vi "校准设置页.vi"() -> ()   [LabVIEW 2016, in "斯坦道总磷.lvlib"]
uses:
  <vilib>/ptbypt/NI_PtbyPt.lvlib
panel:
  in  "校准任务":bool
  in  "历史数据导入":T1(radio)
  out "刷新时间":string
  out "模型刷新":bool
  in  "校准按钮":T1(radio)
  in  "仪器写入":bool
  in  "辅助计算":bool
  in  "曲线模型":T2={"标液浓度1"=0.0, "测量吸光度1"=0.0, "样品1启用"=FALSE, "标液浓度2"=0.0, "测量吸光度2"=0.0, "样品2启用"=FALSE, "标液浓度3"=0.0, "测量吸光度3"=0.0, "样品3启用"=FALSE, "标液浓度4"=0.0, "测量吸光度4"=0.0, "样品4启用"=FALSE, "标液浓度5"=0.0, "测量吸光度5"=0.0, "样品5启用"=FALSE, "模型"=enum."线性", "精度"=4.0, "XY图"=[], "拟合公式"="", "r^2"=0.0, "标样一校准时间"=timestamp(0 s since 1904-01-01), "标样二校准时间"=timestamp(0 s since 1904-01-01), "标样三校准时间"=timestamp(0 s since 1904-01-01), "标样四校准时间"=timestamp(0 s since 1904-01-01), "标样五校准时间"=timestamp(0 s since 1904-01-01), "二次方程"={"c"=0.0, "x"=0.0, "x^2"=0.0}, "标定时间"=timestamp(0 s since 1904-01-01)} {"标定时间" format="%<%y/%m/%d %H:%M:%S>T"; "标样五校准时间" format="%<%y/%m/%d %H:%M:%S>T"; "标样四校准时间" format="%<%y/%m/%d %H:%M:%S>T"; "标样三校准时间" format="%<%y/%m/%d %H:%M:%S>T"; "标样二校准时间" format="%<%y/%m/%d %H:%M:%S>T"; "标样一校准时间" format="%<%y/%m/%d %H:%M:%S>T"; "r^2" format="%.7f"; "测量吸光度5" format="%#.6f"; "测量吸光度4" format="%#.6f"; "测量吸光度3" format="%#.6f"; "测量吸光度2" format="%#.6f"; "测量吸光度1" format="%#.6f"}
  in  "测量模式":T3(ring)
  in  "参数下拉列表":u16(ring)
  in  "量程下拉列表":enum16{"低量程", "高量程"}(ring)
  # "校准时间"
  # "标液浓度"
  # "吸光值"
  # "标样一"
  # "标样二"
  # "标样三"
  # "零点"
  # "跨度"
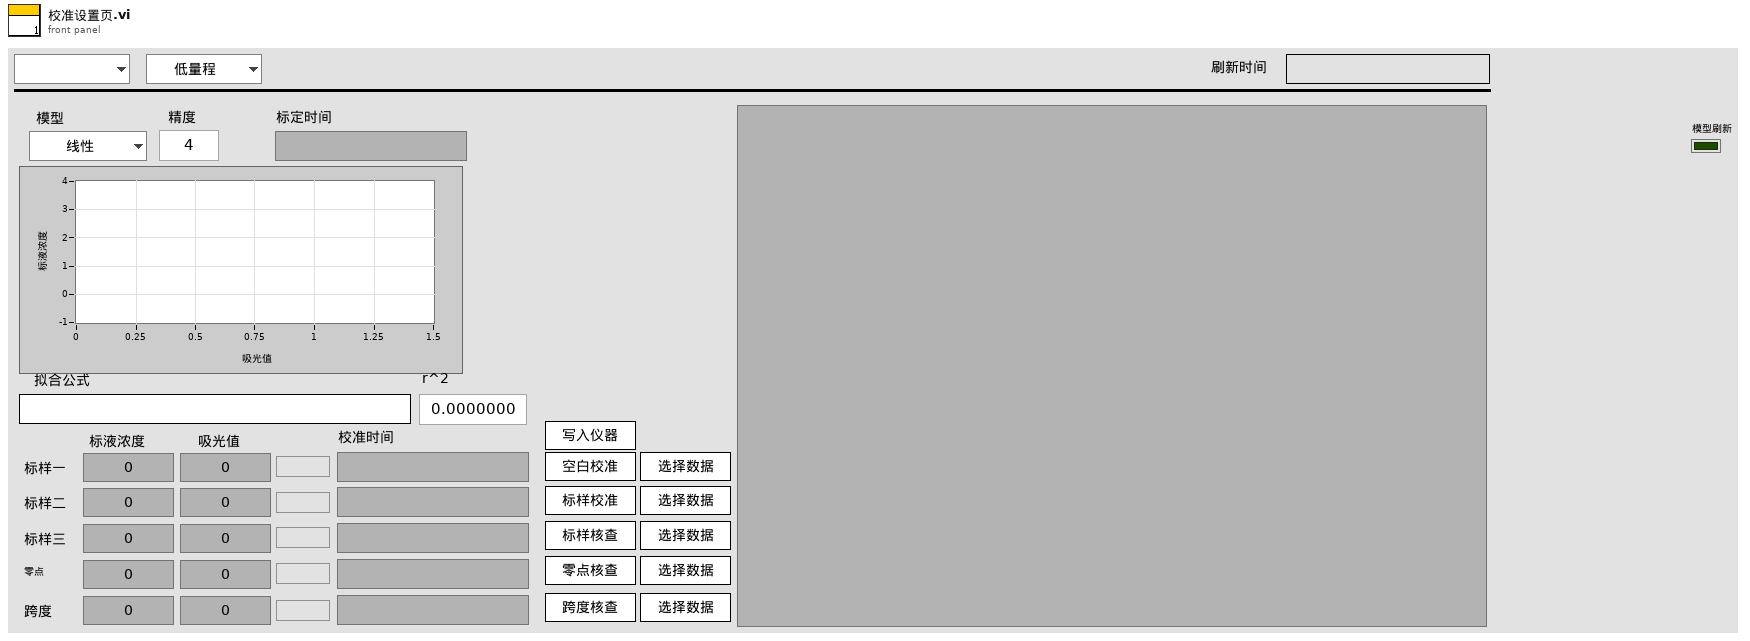
[diagram p1: front panel]
types:
  T1 = enum32{"未选择", "空白校准", "标样校准", "标样核查", "零点核查", "跨度核查"}
  T2 = cluster{"标液浓度1":dbl, "测量吸光度1":dbl, "样品1启用":bool, "标液浓度2":dbl, "测量吸光度2":dbl, "样品2启用":bool, "标液浓度3":dbl, "测量吸光度3":dbl, "样品3启用":bool, "标液浓度4":dbl, "测量吸光度4":dbl, "样品4启用":bool, "标液浓度5":dbl, "测量吸光度5":dbl, "样品5启用":bool, "模型":enum32{"线性", "多项式"}, "精度":dbl, "XY图":cluster{"X Values":dbl[], "Y Values":dbl[]}[], "拟合公式":string, "r^2":dbl, "标样一校准时间":timestamp, "标样二校准时间":timestamp, "标样三校准时间":timestamp, "标样四校准时间":timestamp, "标样五校准时间":timestamp, "二次方程":cluster{"c":dbl, "x":dbl, "x^2":dbl}, "标定时间":timestamp}
  T3 = enum16{"跨度核查", "水样测量", "零点核查", "标样核查", "加标回收", "快捷测试", "空白校准", "标样校准"}
  T4 = typedef "斯坦道总磷.lvlib/校准任务.ctl" = cluster{"id":u16, "任务类型":enum16{"未选择", "空白校准", "标样校准", "标样核查", "零点核查", "跨度核查"}, "量程下拉列表":enum16{"低量程", "高量程"}, "状态":enum16{"已执行", "待执行", "执行中", "停止"}, "标液浓度":dbl, "吸光值":dbl, "校准时间":timestamp}
  T5 = enum8{"Enabled", "Disabled", "Disabled and Grayed Out"}
  T6 = cluster{"低标液1浓度":dbl, "低标液1信号值":dbl, "低标液1启用":u16, "低标液2浓度":dbl, "低标液2信号值":dbl, "低标液2启用":u16, "低标液3浓度":dbl, "低标液3信号值":dbl, "低标液3启用":u16, "低标液4浓度":dbl, "低标液4信号值":dbl, "低标液4启用":u16, "低标液5浓度":dbl, "低标液5信号值":dbl, "低标液5启用":u16, "高标液1浓度":dbl, "高标液1信号值":dbl, "高标液1启用":u16, "高标液2浓度":dbl, "高标液2信号值":dbl, "高标液2启用":u16, "高标液3浓度":dbl, "高标液3信号值":dbl, "高标液3启用":u16, "高标液4浓度":dbl, "高标液4信号值":dbl, "高标液4启用":u16, "高标液5浓度":dbl, "高标液5信号值":dbl, "高标液5启用":u16}
  T7 = cluster{"标液浓度1":dbl, "测量吸光度1":dbl, "样品1启用":bool, "标液浓度2":dbl, "测量吸光度2":dbl, "样品2启用":bool, "标液浓度3":dbl, "测量吸光度3":dbl, "样品3启用":bool, "标液浓度4":dbl, "测量吸光度4":dbl, "样品4启用":bool, "标液浓度5":dbl, "测量吸光度5":dbl, "样品5启用":bool, "模型":enum32{"线性", "多项式"}, "精度":dbl, "XY图":cluster{"X Values":dbl[], "Y Values":dbl[]}[], "拟合公式":string, "r^2":dbl, "标样一校准时间":timestamp, "标样二校准时间":timestamp, "标样三校准时间":timestamp, "标样四校准时间":timestamp, "标样五校准时间":timestamp, "二次方程":cluster{"c":dbl, "x":dbl, "x^2":dbl}, "标定时间":timestamp}[]
  T8 = cluster{"标液浓度1":dbl, "测量吸光度1":dbl, "样品1启用":bool, "标液浓度2":dbl, "测量吸光度2":dbl, "样品2启用":bool, "标液浓度3":dbl, "测量吸光度3":dbl, "样品3启用":bool, "标液浓度4":dbl, "测量吸光度4":dbl, "样品4启用":bool, "标液浓度5":dbl, "测量吸光度5":dbl, "样品5启用":bool, "模型":enum32{"线性", "多项式"}, "精度":dbl, "XY图":cluster{"X Values":dbl[], "Y Values":dbl[]}[], "拟合公式":string, "r^2":dbl, "标样一校准时间":timestamp, "标样二校准时间":timestamp, "标样三校准时间":timestamp, "标样四校准时间":timestamp, "标样五校准时间":timestamp, "二次方程":cluster{"c":dbl, "x":dbl, "x^2":dbl}, "标定时间":timestamp}[][]
  T9 = typedef "LVStringsAndValuesArrayTypeDef_U16.ctl" = cluster{"String":string, "Value":u16}[]
  T10 = cluster{"系统时间":timestamp, "工作状态":u16, "测量模式":enum16{"待机", "连续模式", "周期模式", "定点模式", "受控模式", "手动模式"}, "告警代码":u16, "故障代码":u16, "日志代码":u16, "软件版本":u16, "F0":sgl, "F1":sgl, "F2":sgl, "F3":sgl, "T":sgl, "H":sgl, "id":u16, "flowid":u16, "量程":u16, "总磷控温温度1":sgl, "营养盐控温温度2":sgl, "ADC":sgl}
  T11 = cluster{"时间":timestamp, "标液值":dbl, "检测值":dbl, "吸光值":dbl}
  T12 = enum32{"Bad", "Idle", "Run top level", "Running"}
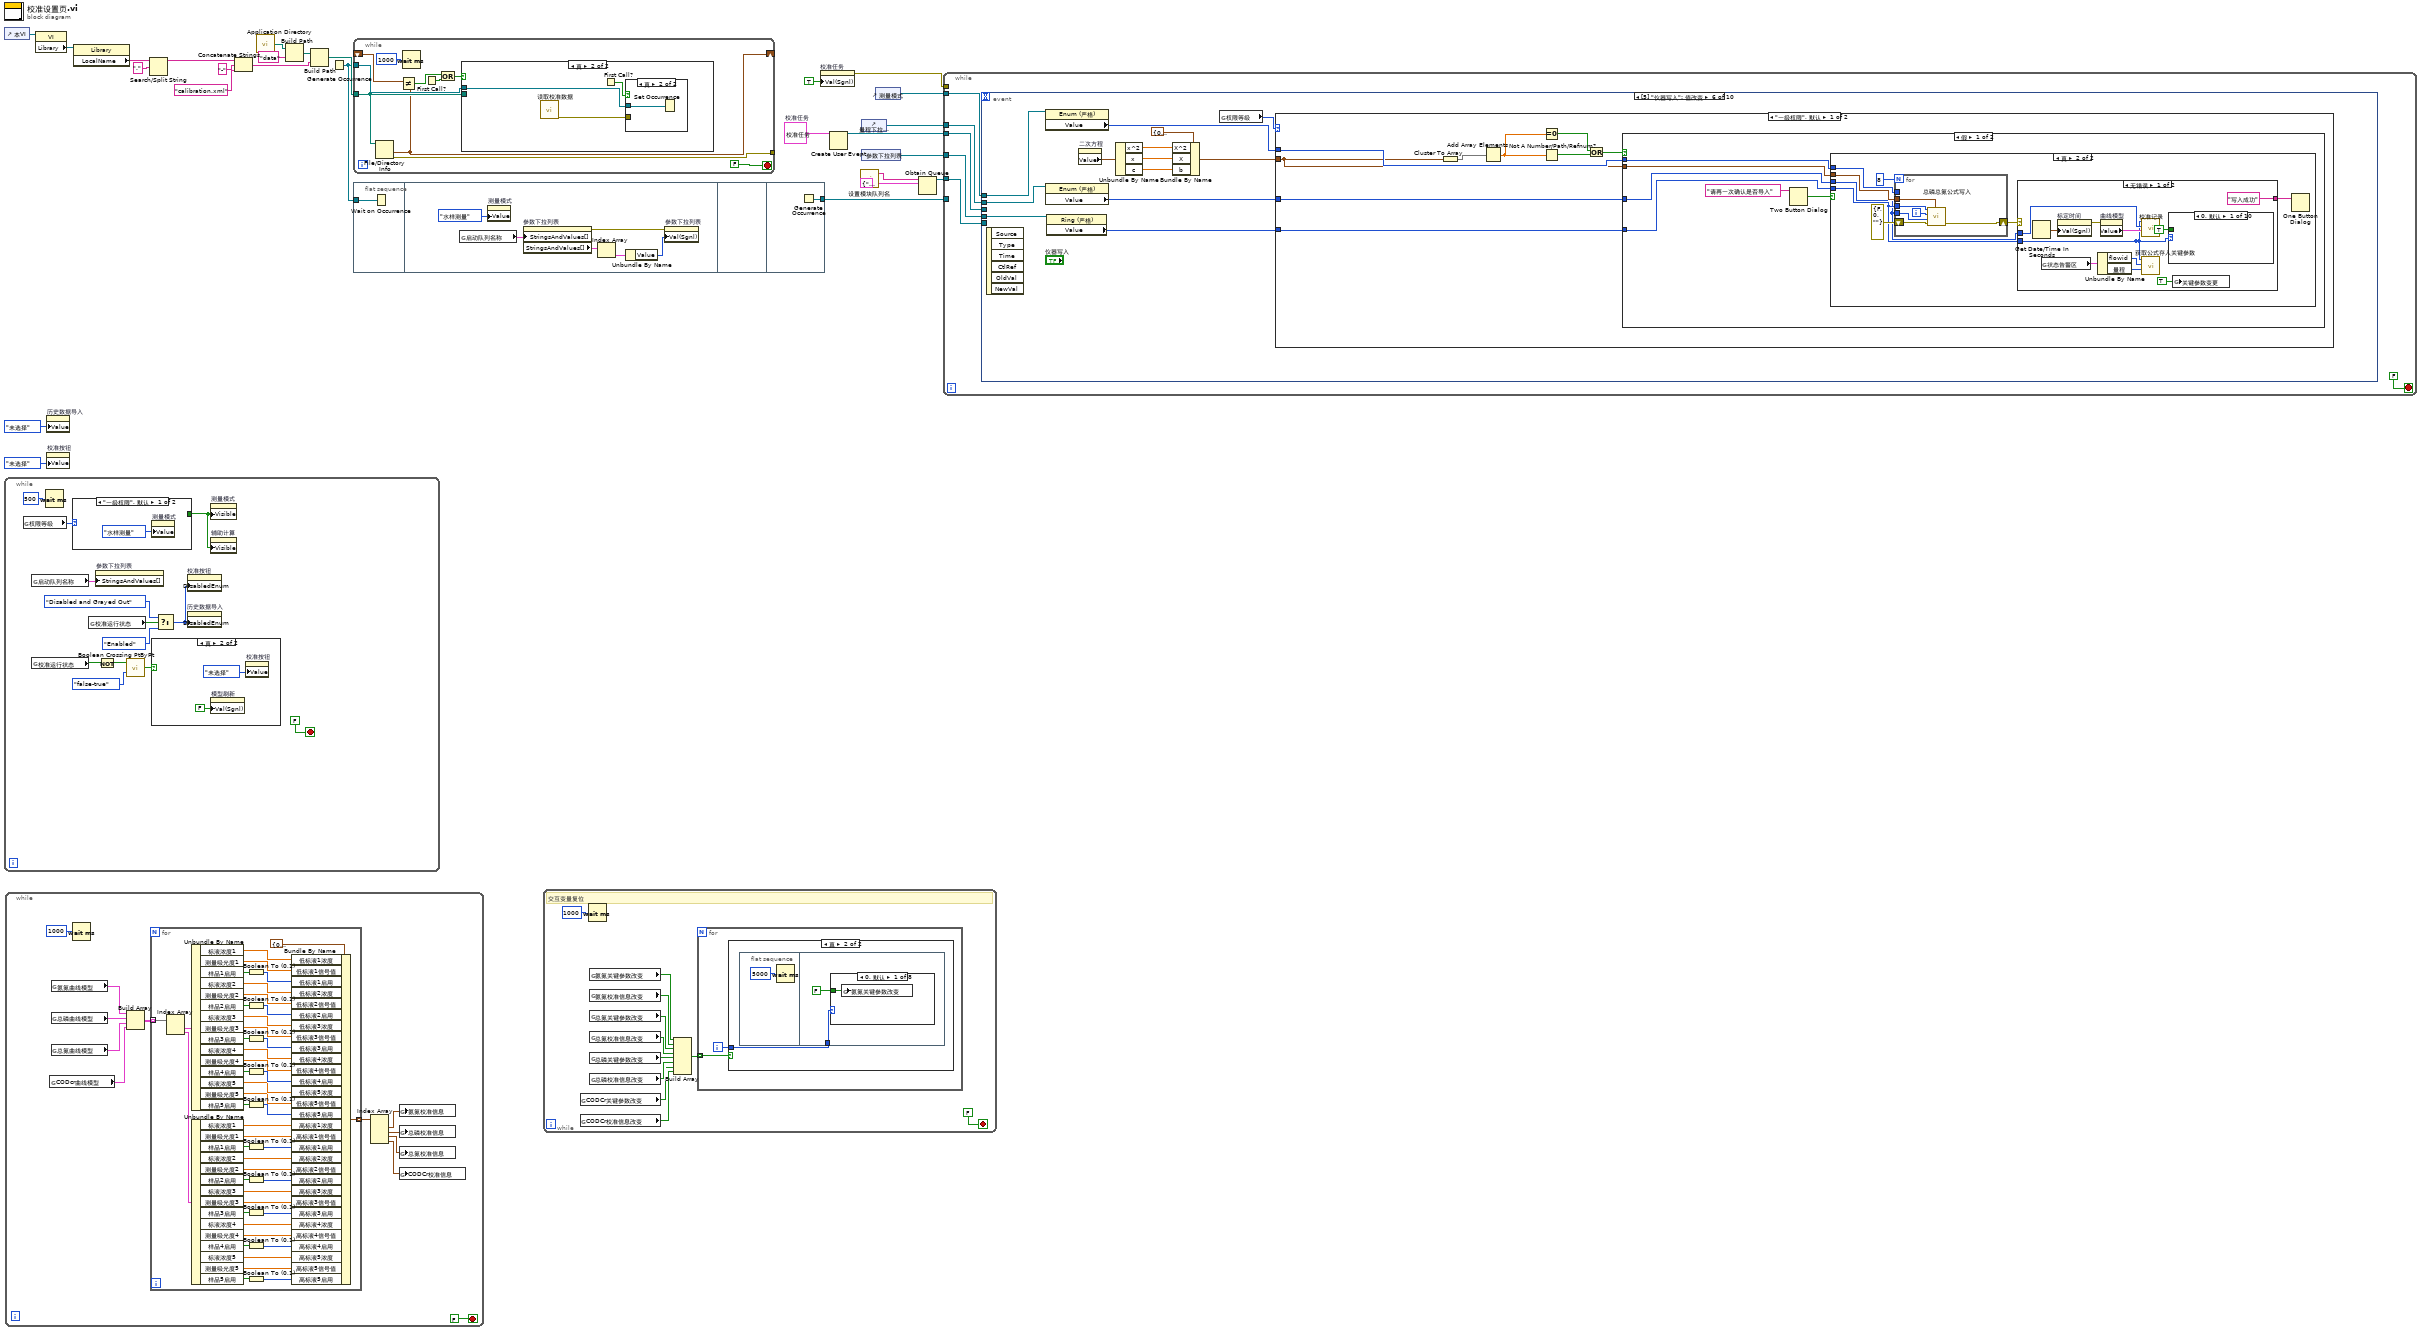
[diagram p0: block diagram]
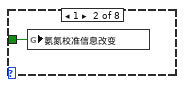
[diagram p3: hidden frame]
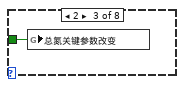
[diagram p4: hidden frame]
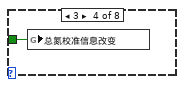
[diagram p5: hidden frame]
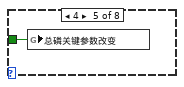
[diagram p6: hidden frame]
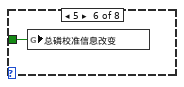
[diagram p7: hidden frame]
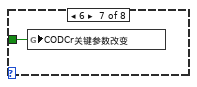
[diagram p8: hidden frame]
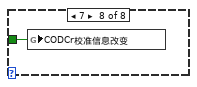
[diagram p9: hidden frame]
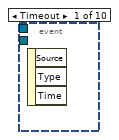
[diagram p12: hidden frame]
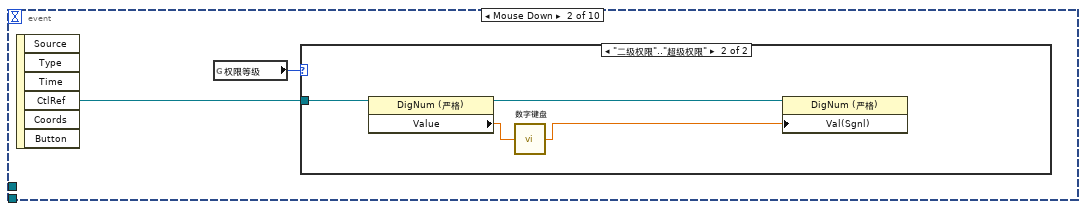
[diagram p13: hidden frame]
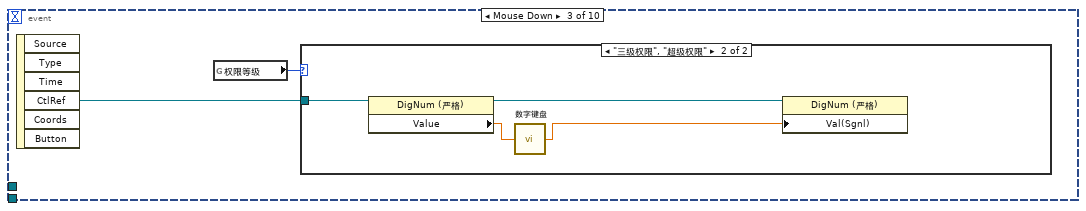
[diagram p15: hidden frame]
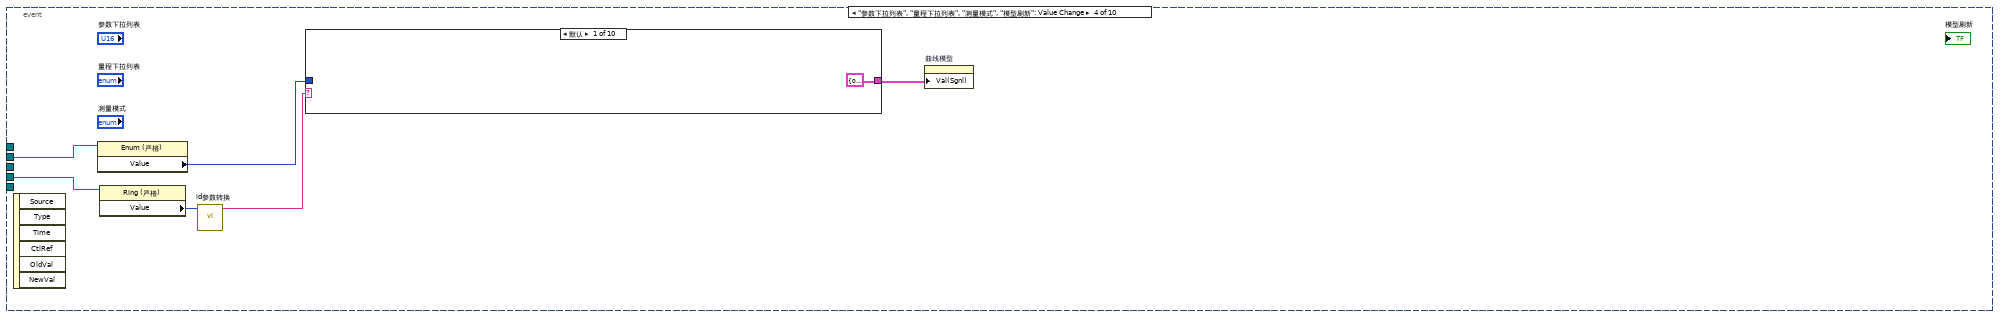
[diagram p17: hidden frame]
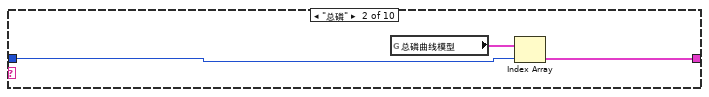
[diagram p18: hidden frame]
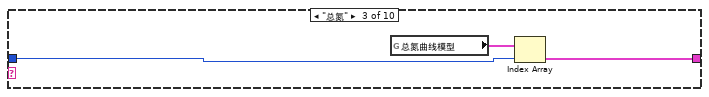
[diagram p19: hidden frame]
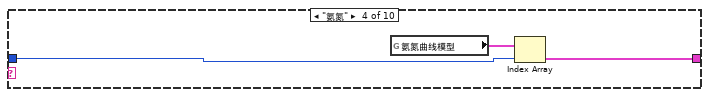
[diagram p20: hidden frame]
diagram:
  w3 = T4 {"id"=1, "任务类型"=enum."未选择", "量程下拉列表"=enum."低量程", "状态"=enum."已执行", "标液浓度"=0.0, "吸光值"=0.0, "校准时间"=timestamp(0 s since 1904-01-01)}  # 校准任务
  n1 = control-ref of="本VI"() -> (w14:refnum<vi>)
  n2 = while {
    stop <- FALSE stop-if-true
    n3 = global read "VAR总磷总氮全局变量.vi" "权限等级"() -> (w37:enum16{"一级权限", "二级权限", "三级权限", "超级权限"})
    n4 = global read "model config var.vi" "启动队列名称"() -> (w34:cluster{"String":string, "Value":u16}[])
    n5 = global read "VAR总磷总氮全局变量.vi" "校准运行状态"() -> (w33:bool)
    n6 = Wait (ms)(milliseconds to wait=u32 500 ("等待时间（毫秒）")) -> ()  [unwired: 1 out]
    n7 = case shown="\"一级权限\", 默认" w37 {
      tunnel: [_ TRUE ("可见")] -> w27
      frame "一级权限", Default {
        n8 = property on="测量模式" class="Enum (严格)"("Value"=T3."水样测量" ("测量模式")) -> ()  [unwired: 2 in, 2 out]
      }
      frame "三级权限", "超级权限" {
      }
    }
    n9 = global read "VAR总磷总氮全局变量.vi" "校准运行状态"() -> (w31:bool)
    n10 = property on="参数下拉列表" class="Ring (严格)"("StringsAndValues[]"=w34) -> ()  [unwired: 2 in, 2 out]
    n11 = Not(x=w33) -> (.not. x?=w32:bool)
    n12 = call <vilib>:"Boolean Crossing PtByPt.vi"("direction"=enum16{"either", "false-true", "true-false"}."false-true", "input"=w32) -> ("crossing"=w35:bool)  [unwired: 1 in]
    n13 = case shown="真" w35 {
      frame False {
      }
      frame True {
        n14 = property on="模型刷新" class="Bool (严格)"("Val(Sgnl)"=FALSE ("值(信号)")) -> ()  [unwired: 2 in, 2 out]
        n15 = property on="校准按钮" class="RadioBtnsControl (严格)"("Value"=T1."未选择" ("校准按钮")) -> ()  [unwired: 2 in, 2 out]
      }
    }
    n16 = Select(t=T5."Disabled and Grayed Out" ("禁用"), s=w31, f=T5."Enabled" ("禁用")) -> (s? t:f=w29:T5)
    n17 = property on="校准按钮" class="RadioBtnsControl (严格)"("DisabledEnum"=w29) -> ()  [unwired: 2 in, 2 out]
    n18 = property on="历史数据导入" class="RadioBtnsControl (严格)"("DisabledEnum"=w29) -> ()  [unwired: 2 in, 2 out]
    n19 = property on="测量模式" class="Enum (严格)"("Visible"=w27) -> ()  [unwired: 2 in, 2 out]
    n20 = property on="辅助计算" class="Bool"("Visible"=w27) -> ()  [unwired: 2 in, 2 out]
  }
  n21 = while {
    stop <- FALSE stop-if-true
    n22 = global read "校准数据全局变量.vi" "CODcr曲线模型"() -> (w52:T7)
    n23 = global read "校准数据全局变量.vi" "氨氮曲线模型"() -> (w55:T7)
    n24 = global read "校准数据全局变量.vi" "总磷曲线模型"() -> (w54:T7)
    n25 = global read "校准数据全局变量.vi" "总氮曲线模型"() -> (w53:T7)
    n26 = Wait (ms)(milliseconds to wait=u32 1000 ("等待时间（毫秒）")) -> ()  [unwired: 1 out]
    n27 = Build Array(w55, w54, w53, w52) -> (w51:T8)
    n28 = for {
      tunnel: [w100] -> w50 mode=indexing
      tunnel: w51 -> [w57] mode=indexing
      n29 = Index Array(array=w57) -> (element #1=w99:T2, element #2=w96:T2)  [unwired: 2 in]
      n30 = Unbundle By Name(w99) -> ("标液浓度1"=w84:dbl, "测量吸光度1"=w83:dbl, "样品1启用"=w98:bool, "标液浓度2"=w82:dbl, "测量吸光度2"=w81:dbl, "样品2启用"=w93:bool, "标液浓度3"=w63:dbl, "测量吸光度3"=w62:dbl, "样品3启用"=w92:bool, "标液浓度4"=w61:dbl, "测量吸光度4"=w60:dbl, "样品4启用"=w91:bool, "标液浓度5"=w59:dbl, "测量吸光度5"=w58:dbl, "样品5启用"=w90:bool)
      n31 = Unbundle By Name(w96) -> ("标液浓度1"=w95:dbl, "测量吸光度1"=w94:dbl, "样品1启用"=w89:bool, "标液浓度2"=w71:dbl, "测量吸光度2"=w70:dbl, "样品2启用"=w88:bool, "标液浓度3"=w69:dbl, "测量吸光度3"=w68:dbl, "样品3启用"=w87:bool, "标液浓度4"=w67:dbl, "测量吸光度4"=w66:dbl, "样品4启用"=w86:bool, "标液浓度5"=w65:dbl, "测量吸光度5"=w64:dbl, "样品5启用"=w85:bool)
      n32 = Boolean To (0,1)(Boolean=w98) -> (0, 1=w97:i16)
      n33 = Boolean To (0,1)(Boolean=w93) -> (0, 1=w80:i16)
      n34 = Boolean To (0,1)(Boolean=w92) -> (0, 1=w79:i16)
      n35 = Boolean To (0,1)(Boolean=w91) -> (0, 1=w78:i16)
      n36 = Boolean To (0,1)(Boolean=w90) -> (0, 1=w77:i16)
      n37 = Boolean To (0,1)(Boolean=w89) -> (0, 1=w76:i16)
      n38 = Boolean To (0,1)(Boolean=w88) -> (0, 1=w75:i16)
      n39 = Boolean To (0,1)(Boolean=w87) -> (0, 1=w74:i16)
      n40 = Boolean To (0,1)(Boolean=w86) -> (0, 1=w73:i16)
      n41 = Boolean To (0,1)(Boolean=w85) -> (0, 1=w72:i16)
      n42 = Bundle By Name(cluster=T6 {"低标液1浓度"=0.0, "低标液1信号值"=0.0, "低标液1启用"=0, "低标液2浓度"=0.0, "低标液2信号值"=0.0, "低标液2启用"=0, "低标液3浓度"=0.0, "低标液3信号值"=0.0, "低标液3启用"=0, "低标液4浓度"=0.0, "低标液4信号值"=0.0, "低标液4启用"=0, "低标液5浓度"=0.0, "低标液5信号值"=0.0, "低标液5启用"=0, "高标液1浓度"=0.0, "高标液1信号值"=0.0, "高标液1启用"=0, "高标液2浓度"=0.0, "高标液2信号值"=0.0, "高标液2启用"=0, "高标液3浓度"=0.0, "高标液3信号值"=0.0, "高标液3启用"=0, "高标液4浓度"=0.0, "高标液4信号值"=0.0, "高标液4启用"=0, "高标液5浓度"=0.0, "高标液5信号值"=0.0, "高标液5启用"=0} ("氨氮校准信息"), "低标液1浓度"=w84, "低标液1信号值"=w83, "低标液1启用"=w97, "低标液2浓度"=w82, "低标液2信号值"=w81, "低标液2启用"=w80, "低标液3浓度"=w63, "低标液3信号值"=w62, "低标液3启用"=w79, "低标液4浓度"=w61, "低标液4信号值"=w60, "低标液4启用"=w78, "低标液5浓度"=w59, "低标液5信号值"=w58, "低标液5启用"=w77, "高标液1浓度"=w95, "高标液1信号值"=w94, "高标液1启用"=w76, "高标液2浓度"=w71, "高标液2信号值"=w70, "高标液2启用"=w75, "高标液3浓度"=w69, "高标液3信号值"=w68, "高标液3启用"=w74, "高标液4浓度"=w67, "高标液4信号值"=w66, "高标液4启用"=w73, "高标液5浓度"=w65, "高标液5信号值"=w64, "高标液5启用"=w72) -> (w100:T6)
    }
    n43 = Index Array(array=w50) -> (element #1=w49:T6, element #2=w48:T6, element #3=w47:T6, element #4=w46:T6)  [unwired: 4 in]
    n44 = global write "VAR总磷总氮全局变量.vi" "氨氮校准信息"(w49) -> ()
    n45 = global write "VAR总磷总氮全局变量.vi" "总磷校准信息"(w48) -> ()
    n46 = global write "VAR总磷总氮全局变量.vi" "总氮校准信息"(w47) -> ()
    n47 = global write "VAR总磷总氮全局变量.vi" "CODCr校准信息"(w46) -> ()
  }
  n48 = property class="VI"(reference=w14) -> ("Library"=w15:refnum<vi>)  [unwired: 1 in, 2 out]
  n49 = property on="历史数据导入" class="RadioBtnsControl (严格)"("Value"=T1."未选择" ("历史数据导入")) -> ()  [unwired: 2 in, 2 out]
  n50 = property on="校准按钮" class="RadioBtnsControl (严格)"("Value"=T1."未选择" ("校准按钮")) -> ()  [unwired: 2 in, 2 out]
  n51 = property class="Library"(reference=w15) -> ("LocalName"=w12:string)  [unwired: 1 in, 2 out]
  n52 = Search/Split String(string=w12, search string/char (-)="." ("搜索字符串/字符(-)")) -> (substring before match=w10:string)  [unwired: 1 in, 2 out]
  n53 = Concatenate Strings(w10, "-" ("字符串"), "calibration.xml" ("名称或相对路径")) -> (w7:string)
  n54 = call <vilib>:"Application Directory.vi"() -> ("Application Directory"=w16:path)
  n55 = Build Path(base path=w16, name or relative path="data" ("名称或相对路径")) -> (appended path=w13:path)
  n56 = Build Path(base path=w13, name or relative path=w7) -> (appended path=w6:path)
  n57 = Generate Occurrence() -> (w5:refnum<k4>)
  n58 = while {
    shift-right: [w101] -> _
    shift-left: _ -> [w109]
    tunnel: w6 -> [w107]
    tunnel: [w105] -> _
    tunnel: w5 -> [w104]
    stop <- FALSE stop-if-true
    n59 = File/Directory Info(path=w107) -> (last mod=w101:timestamp, error out=w105:errorcluster)  [unwired: 1 in, 5 out]
    n60 = Not Equal?(x=w109, y=w101) -> (x != y?=w108:bool)
    n61 = Wait (ms)(milliseconds to wait=u32 1000 ("等待时间（毫秒）")) -> ()  [unwired: 1 out]
    n62 = First Call?() -> (First Call?: T/F=w102:bool)
    n63 = Or(x=w108, y=w102) -> (x .or. y?=w103:bool)
    n64 = case shown="真" w103 {
      tunnel: w107 -> [_ _]
      tunnel: w104 -> [_ w113]
      frame False {
      }
      frame True {
        n65 = call "读取校准数据.vi"() -> ("错误输出"=w112:errorcluster)  [unwired: 11 in]
        n66 = First Call?() -> (First Call?: T/F=w111:bool)
        n67 = case shown="真" w111 {
          tunnel: w113 -> [_ w114]
          tunnel: w112 -> [_ _]
          frame False {
          }
          frame True {
            n68 = Set Occurrence(w114) -> ()
          }
        }
      }
    }
  }
  n69 = flat-sequence {
    tunnel: w5 -> [w115]
    tunnel: [w122] -> w26
    frame #0 {
      n70 = Wait on Occurrence(2:w115) -> ()  [unwired: 2 in, 1 out]
    }
    frame #1 {
      n71 = global read "model config var.vi" "启动队列名称"() -> (w117:cluster{"String":string, "Value":u16}[])
      n72 = property on="测量模式" class="Enum (严格)"("Value"=T3."水样测量" ("测量模式")) -> ()  [unwired: 2 in, 2 out]
      n73 = property on="参数下拉列表" class="Ring (严格)"("StringsAndValues[]"=w117) -> (error out=w120:errorcluster, "StringsAndValues[]"=w118:T9)  [unwired: 2 in, 1 out]
      n74 = Index Array(array=w118) -> (element=w119:cluster{"String":string, "Value":u16})  [unwired: 1 in]
      n75 = Unbundle By Name(w119) -> ("Value"=w121:u16)
      n76 = property on="参数下拉列表" class="Ring (严格)"(error in=w120, "Val(Sgnl)"=w121) -> ()  [unwired: 1 in, 2 out]
    }
    frame #2 {
    }
    frame #3 {
      n77 = Generate Occurrence() -> (w122:refnum<k4>)
    }
  }
  n78 = while {
    stop <- FALSE stop-if-true
    # "交互变量复位"
    n79 = global read "VAR总磷总氮全局变量.vi" "CODCr关键参数改变"() -> (w127:bool)
    n80 = global read "VAR总磷总氮全局变量.vi" "CODCr校准信息改变"() -> (w126:bool)
    n81 = Wait (ms)(milliseconds to wait=u32 1000 ("等待时间（毫秒）")) -> ()  [unwired: 1 out]
    n82 = global read "VAR总磷总氮全局变量.vi" "氨氮关键参数改变"() -> (w133:bool)
    n83 = global read "VAR总磷总氮全局变量.vi" "氨氮校准信息改变"() -> (w132:bool)
    n84 = global read "VAR总磷总氮全局变量.vi" "总氮关键参数改变"() -> (w131:bool)
    n85 = global read "VAR总磷总氮全局变量.vi" "总氮校准信息改变"() -> (w130:bool)
    n86 = global read "VAR总磷总氮全局变量.vi" "总磷关键参数改变"() -> (w129:bool)
    n87 = global read "VAR总磷总氮全局变量.vi" "总磷校准信息改变"() -> (w128:bool)
    n88 = Build Array(w133, w132, w131, w130, w129, w128, w127, w126) -> (w125:bool[])
    n89 = for {
      tunnel: w125 -> [w135] mode=indexing
      i -> [w134]
      n90 = case shown="真" w135 {
        tunnel: w134 -> [_ w136]
        frame False {
        }
        frame True {
          n91 = flat-sequence {
            tunnel: w136 -> [w139]
            frame #0 {
              n92 = Wait (ms)(milliseconds to wait=u32 5000 ("等待时间（毫秒）")) -> ()  [unwired: 1 out]
            }
            frame #1 {
              n93 = case shown="0, 默认" w139 {
                tunnel: FALSE -> [w140 w141 w142 w143 w144 w145 w146 w147]
                frame 0, Default {
                  n94 = global write "VAR总磷总氮全局变量.vi" "氨氮关键参数改变"(w140) -> ()
                }
                frame 1 {
                  n95 = global write "VAR总磷总氮全局变量.vi" "氨氮校准信息改变"(w141) -> ()
                }
                frame 2 {
                  n96 = global write "VAR总磷总氮全局变量.vi" "总氮关键参数改变"(w142) -> ()
                }
                frame 3 {
                  n97 = global write "VAR总磷总氮全局变量.vi" "总氮校准信息改变"(w143) -> ()
                }
                frame 4 {
                  n98 = global write "VAR总磷总氮全局变量.vi" "总磷关键参数改变"(w144) -> ()
                }
                frame 5 {
                  n99 = global write "VAR总磷总氮全局变量.vi" "总磷校准信息改变"(w145) -> ()
                }
                frame 6 {
                  n100 = global write "VAR总磷总氮全局变量.vi" "CODCr关键参数改变"(w146) -> ()
                }
                frame 7 {
                  n101 = global write "VAR总磷总氮全局变量.vi" "CODCr校准信息改变"(w147) -> ()
                }
              }
            }
          }
        }
      }
    }
  }
  n102 = property on="校准任务" class="Bool (严格)"("Val(Sgnl)"=TRUE ("值(信号)")) -> (error out=w2:errorcluster)  [unwired: 2 in, 1 out]
  n103 = Create User Event(user event datatype=w3) -> (user event=w4:refnum<user-event>)  [unwired: 1 in, 1 out]
  n104 = call "设置模块队列名.vi"() -> ("Msg"=w24:string)  [unwired: 5 in]
  n105 = control-ref of="量程下拉列表"() -> (w19:refnum<vi>)
  n106 = control-ref of="参数下拉列表"() -> (w21:refnum<vi>)
  n107 = control-ref of="测量模式"() -> (w20:refnum<vi>)
  n108 = Obtain Queue(name (unnamed)=w24, element data type=cluster{"命令":string, "data":variant} {"命令"="", "data"=variant}) -> (queue out=w23:refnum<queue>)  [unwired: 3 in, 2 out]
  n109 = while {
    tunnel: w26 -> [_]
    tunnel: w21 -> [w152]
    tunnel: w20 -> [w151]
    tunnel: w19 -> [w150]
    tunnel: w23 -> [w149]
    tunnel: w4 -> [w148]
    tunnel: w2 -> [_]
    stop <- FALSE stop-if-true
    n110 = event shown="[5] \"仪器写入\": 值改变" {
      selector: _ -> [_ _ _ _ _ _ _ _ _ _]
      dyn-events: _ -> [_ _ _ _ _ _ _ _ _ _]
      timeout: _ -> [_ _ _ _ _ _ _ _ _ _]
      tunnel: w152 -> [_ _ _ w170 _ w225 w279 w333 w361 _]
      tunnel: w151 -> [_ _ _ _ _ w223 _ w328 w356 _]
      tunnel: w150 -> [_ _ _ w168 _ w221 w277 w332 w360 _]
      tunnel: w149 -> [_ _ _ _ _ _ _ w334 w362 _]
      tunnel: w148 -> [_ _ _ _ _ _ _ w327 w355 w384]
      event Timeout {
        n111 = event-data() -> ()  [unwired: 1 in, 3 out]
      }
      event "曲线模型.标液浓度1", "曲线模型.标液浓度2", "曲线模型.标液浓度3", "曲线模型.标液浓度4", "曲线模型.标液浓度5", "曲线模型.精度": Mouse Down {
        n112 = event-data() -> ("CtlRef"=w155:refnum<vi>)  [unwired: 1 in, 5 out]
        n113 = global read "VAR总磷总氮全局变量.vi" "权限等级"() -> (w154:enum16{"一级权限", "二级权限", "三级权限", "超级权限"})
        n114 = case shown="\"二级权限\"..\"超级权限\"" w154 {
          tunnel: w155 -> [_ w159]
          frame "一级权限", Default {
          }
          frame "二级权限".."超级权限" {
            n115 = property class="DigNum (严格)"(reference=w159) -> (reference out=w157:refnum<vi>, "Value"=w158:dbl)  [unwired: 1 in, 1 out]
            n116 = call "数字键盘.vi"("OldNumber"=w158) -> ("NewNumber"=w156:dbl)
            n117 = property class="DigNum (严格)"(reference=w157, "Val(Sgnl)"=w156) -> ()  [unwired: 1 in, 2 out]
          }
        }
      }
      event "曲线模型.测量吸光度1", "曲线模型.测量吸光度2", "曲线模型.测量吸光度3", "曲线模型.测量吸光度4", "曲线模型.测量吸光度5": Mouse Down {
        n118 = event-data() -> ("CtlRef"=w161:refnum<vi>)  [unwired: 1 in, 5 out]
        n119 = global read "VAR总磷总氮全局变量.vi" "权限等级"() -> (w160:enum16{"一级权限", "二级权限", "三级权限", "超级权限"})
        n120 = case shown="\"三级权限\", \"超级权限\"" w160 {
          tunnel: w161 -> [_ w165]
          frame "一级权限", Default {
          }
          frame "三级权限", "超级权限" {
            n121 = property class="DigNum (严格)"(reference=w165) -> (reference out=w163:refnum<vi>, "Value"=w164:dbl)  [unwired: 1 in, 1 out]
            n122 = call "数字键盘.vi"("OldNumber"=w164) -> ("NewNumber"=w162:dbl)
            n123 = property class="DigNum (严格)"(reference=w163, "Val(Sgnl)"=w162) -> ()  [unwired: 1 in, 2 out]
          }
        }
      }
      event "参数下拉列表", "量程下拉列表", "测量模式", "模型刷新": Value Change {
        n124 = event-data() -> ()  [unwired: 1 in, 6 out]
        n125 = property class="Enum (严格)"(reference=w168) -> ("Value"=w166:enum16{"低量程", "高量程"})  [unwired: 1 in, 2 out]
        n126 = property class="Ring (严格)"(reference=w170) -> ("Value"=w171:u16)  [unwired: 1 in, 2 out]
        n127 = call "id参数转换.vi"("id"=w171) -> ("table输出"=w169:string)  [unwired: 9 in, 1 out]
        n128 = case shown="默认" w169 {
          tunnel: w166 -> [_ w173 w176 w179 w182 w185 w188 w191 w194 w197]
          tunnel: [T2 {"标液浓度1"=0.0, "测量吸光度1"=0.0, "样品1启用"=FALSE, "标液浓度2"=0.0, "测量吸光度2"=0.0, "样品2启用"=FALSE, "标液浓度3"=0.0, "测量吸光度3"=0.0, "样品3启用"=FALSE, "标液浓度4"=0.0, "测量吸光度4"=0.0, "样品4启用"=FALSE, "标液浓度5"=0.0, "测量吸光度5"=0.0, "样品5启用"=FALSE, "模型"=enum."线性", "精度"=0.0, "XY图"=[], "拟合公式"="", "r^2"=0.0, "标样一校准时间"=timestamp(0 s since 1904-01-01), "标样二校准时间"=timestamp(0 s since 1904-01-01), "标样三校准时间"=timestamp(0 s since 1904-01-01), "标样四校准时间"=timestamp(0 s since 1904-01-01), "标样五校准时间"=timestamp(0 s since 1904-01-01), "二次方程"={"c"=0.0, "x"=0.0, "x^2"=0.0}, "标定时间"=timestamp(0 s since 1904-01-01)} ("总磷曲线模型") w174 w177 w180 w183 w186 w189 w192 w195 w198] -> w167
          frame Default {
          }
          frame "总磷" {
            n129 = global read "校准数据全局变量.vi" "总磷曲线模型"() -> (w175:T7)
            n130 = Index Array(array=w175, index=w173) -> (element=w174:T2)
          }
          frame "总氮" {
            n131 = global read "校准数据全局变量.vi" "总氮曲线模型"() -> (w178:T7)
            n132 = Index Array(array=w178, index=w176) -> (element=w177:T2)
          }
          frame "氨氮" {
            n133 = global read "校准数据全局变量.vi" "氨氮曲线模型"() -> (w181:T7)
            n134 = Index Array(array=w181, index=w179) -> (element=w180:T2)
          }
          frame "磷酸盐" {
            n135 = global read "校准数据全局变量.vi" "磷酸盐曲线模型"() -> (w184:T7)
            n136 = Index Array(array=w184, index=w182) -> (element=w183:T2)
          }
          frame "硝氮" {
            n137 = global read "校准数据全局变量.vi" "硝氮曲线模型"() -> (w187:T7)
            n138 = Index Array(array=w187, index=w185) -> (element=w186:T2)
          }
          frame "亚硝氮" {
            n139 = global read "校准数据全局变量.vi" "亚硝氮曲线模型"() -> (w190:T7)
            n140 = Index Array(array=w190, index=w188) -> (element=w189:T2)
          }
          frame "硅酸盐" {
            n141 = global read "校准数据全局变量.vi" "硅酸盐曲线模型"() -> (w193:T7)
            n142 = Index Array(array=w193, index=w191) -> (element=w192:T2)
          }
          frame "硫化物" {
            n143 = global read "校准数据全局变量.vi" "硫化物曲线模型"() -> (w196:T7)
            n144 = Index Array(array=w196, index=w194) -> (element=w195:T2)
          }
          frame "CODcr" {
            n145 = global read "校准数据全局变量.vi" "CODcr曲线模型"() -> (w199:T7)
            n146 = Index Array(array=w199, index=w197) -> (element=w198:T2)
          }
        }
        n147 = property on="曲线模型" class="Clust (严格)"("Val(Sgnl)"=w167) -> ()  [unwired: 2 in, 2 out]
      }
      event "辅助计算": Value Change {
        n148 = event-data() -> ()  [unwired: 1 in, 6 out]
        n149 = call "吸光值辅助计算.vi"() -> ("X"=w201:dbl, "吸光值导出"=w202:u16)  [unwired: 10 in]
        n150 = Get Date/Time In Seconds() -> (seconds since 1Jan1904=w200:timestamp)
        n151 = case shown="4" w202 {
          tunnel: w201 -> [_ w204 w206 w208 w210 w212]
          tunnel: w200 -> [_ w203 w205 w207 w209 w211]
          frame 0, Default {
          }
          frame 1 {
            n152 = property on="标样一校准时间" class="AbsTime (严格)"("Val(Sgnl)"=w203) -> ()  [unwired: 2 in, 2 out]
            n153 = property on="测量吸光度1" class="DigNum (严格)"("Value"=w204) -> ()  [unwired: 2 in, 2 out]
          }
          frame 2 {
            n154 = property on="标样二校准时间" class="AbsTime (严格)"("Val(Sgnl)"=w205) -> ()  [unwired: 2 in, 2 out]
            n155 = property on="测量吸光度2" class="DigNum (严格)"("Value"=w206) -> ()  [unwired: 2 in, 2 out]
          }
          frame 3 {
            n156 = property on="标样三校准时间" class="AbsTime (严格)"("Val(Sgnl)"=w207) -> ()  [unwired: 2 in, 2 out]
            n157 = property on="测量吸光度3" class="DigNum (严格)"("Value"=w208) -> ()  [unwired: 2 in, 2 out]
          }
          frame 4 {
            n158 = property on="标样四校准时间" class="AbsTime (严格)"("Val(Sgnl)"=w209) -> ()  [unwired: 2 in, 2 out]
            n159 = property on="测量吸光度4" class="DigNum (严格)"("Value"=w210) -> ()  [unwired: 2 in, 2 out]
          }
          frame 5 {
            n160 = property on="标样五校准时间" class="AbsTime (严格)"("Val(Sgnl)"=w211) -> ()  [unwired: 2 in, 2 out]
            n161 = property on="测量吸光度5" class="DigNum (严格)"("Value"=w212) -> ()  [unwired: 2 in, 2 out]
          }
        }
      }
      event "仪器写入": Value Change {
        n162 = event-data() -> ()  [unwired: 1 in, 6 out]
        n163 = property class="Enum (严格)"(reference=w223) -> ("Value"=w222:T3)  [unwired: 1 in, 2 out]
        n164 = property class="Enum (严格)"(reference=w221) -> ("Value"=w220:enum16{"低量程", "高量程"})  [unwired: 1 in, 2 out]
        n165 = property class="Ring (严格)"(reference=w225) -> ("Value"=w224:u16)  [unwired: 1 in, 2 out]
        n166 = property on="二次方程" class="Clust (严格)"() -> ("Value"=w214:cluster{"c":dbl, "x":dbl, "x^2":dbl})  [unwired: 2 in, 2 out]
        n167 = Unbundle By Name(w214) -> ("x^2"=w216:dbl, "x"=w217:dbl, "c"=w218:dbl)
        n168 = Bundle By Name(cluster=cluster{"X^2":dbl, "X":dbl, "b":dbl} {"X^2"=0.0, "X"=0.0, "b"=0.0} ("公式"), "X^2"=w216, "X"=w217, "b"=w218) -> (w213:cluster{"X^2":dbl, "X":dbl, "b":dbl})
        n169 = global read "VAR总磷总氮全局变量.vi" "权限等级"() -> (w219:enum16{"一级权限", "二级权限", "三级权限", "超级权限"})
        n170 = case shown="\"一级权限\", 默认" w219 {
          tunnel: w224 -> [w234 w275]
          tunnel: w222 -> [w233 w274]
          tunnel: w220 -> [w232 w273]
          tunnel: w213 -> [w226 w272]
          frame "一级权限", Default {
            n171 = Cluster To Array(cluster=w226) -> (array=w231:dbl[])
            n172 = Add Array Elements(numeric array=w231) -> (sum=w230:dbl)
            n173 = Equal To 0?(x=w230) -> (x = 0?=w228:bool)
            n174 = Not A Number/Path/Refnum?(number/path/refnum=w230) -> (NaN/Path/Refnum?=w229:bool)
            n175 = Or(x=w228, y=w229) -> (x .or. y?=w227:bool)
            n176 = case shown="假" w227 {
              tunnel: w234 -> [w240 _]
              tunnel: w233 -> [w239 _]
              tunnel: w232 -> [w238 _]
              tunnel: w226 -> [w235 _]
              frame False {
                n177 = Two Button Dialog(message="请再一次确认是否导入" ("消息")) -> (T button?=w236:bool)  [unwired: 2 in]
                n178 = case shown="真" w236 {
                  tunnel: w240 -> [_ w242]
                  tunnel: w239 -> [_ w248]
                  tunnel: w238 -> [_ w241]
                  tunnel: w235 -> [_ w243]
                  frame False {
                  }
                  frame True {
                    n179 = for {
                      N: 8 -> [_]
                      tunnel: w242 -> [w254]
                      tunnel: w248 -> [_]
                      tunnel: w241 -> [w253]
                      shift-right: [w252] -> w246
                      shift-left: errorcluster {"status"=FALSE, "code"=0, "source"=""} ("error out") -> [w249]
                      tunnel: w243 -> [w250]
                      i -> [w251]
                      n180 = call "总磷总氮公式写入.vi"("公式"=w250, "error in (no error)"=w249, "量程"=w253, "测量模式"=w251, "测量参数"=w254) -> ("error out"=w252:errorcluster)  [unwired: 6 in]
                    }
                    n181 = case shown="无错误" w246 {
                      tunnel: ["写入成功" "写入失败"] -> w247
                      tunnel: w242 -> [w255 _]
                      tunnel: w241 -> [w263 _]
                      frame No Error {
                        n182 = Get Date/Time In Seconds() -> (seconds since 1Jan1904=w264:timestamp)
                        n183 = global read "VAR总磷总氮全局变量.vi" "状态告警区"() -> (w260:T10)
                        n184 = property on="标定时间" class="AbsTime (严格)"("Val(Sgnl)"=w264) -> (error out=w261:errorcluster)  [unwired: 2 in, 1 out]
                        n185 = Unbundle By Name(w260) -> ("flowid"=w258:u16, "量程"=w259:u16)
                        n186 = property on="曲线模型" class="Clust (严格)"(error in=w261) -> ("Value"=w262:T2)  [unwired: 1 in, 2 out]
                        n187 = call "校准记录.vi"("曲线模型"=w262, "量程"=w263, "校准参数"=w255) -> ()  [unwired: 8 in, 1 out]
                        n188 = call "获取公式存入关键参数.vi"("量程"=w259, "flowid"=w258, "id"=w255) -> ()  [unwired: 8 in, 1 out]
                        n189 = case shown="0, 默认" w255 {
                          tunnel: TRUE ("总磷关键参数改变") -> [_ w266 w267 w268 _ _ _ _ _ w269]
                          frame 0, Default {
                          }
                          frame 1 {
                            n190 = global write "VAR总磷总氮全局变量.vi" "总磷校准信息改变"(w266) -> ()
                          }
                          frame 2 {
                            n191 = global write "VAR总磷总氮全局变量.vi" "总氮校准信息改变"(w267) -> ()
                          }
                          frame 3 {
                            n192 = global write "VAR总磷总氮全局变量.vi" "氨氮校准信息改变"(w268) -> ()
                          }
                          frame 4 {
                          }
                          frame 5 {
                          }
                          frame 6 {
                          }
                          frame 7 {
                          }
                          frame 8 {
                          }
                          frame 22 {
                            n193 = global write "VAR总磷总氮全局变量.vi" "CODCr校准信息改变"(w269) -> ()
                          }
                        }
                        n194 = global write "VAR总磷总氮全局变量.vi" "关键参数变更"(TRUE ("关键参数变更")) -> ()
                      }
                      frame Error {
                      }
                    }
                    n195 = One Button Dialog(message=w247) -> ()  [unwired: 1 in, 1 out]
                  }
                }
              }
              frame True {
                n196 = One Button Dialog(message="校准数据异常，请重新校准！" ("消息")) -> ()  [unwired: 1 in, 1 out]
              }
            }
          }
          frame "三级权限", "超级权限" {
            n197 = call "公式复合写入.vi"("公式"=w272, "量程下拉列表"=w273, "测量模式"=w274, "参数下拉列表"=w275) -> ()  [unwired: 8 in]
          }
        }
      }
      event "曲线模型": Value Change {
        n198 = event-data() -> ()  [unwired: 1 in, 6 out]
        n199 = flat-sequence {
          tunnel: [w284] -> w280
          tunnel: w279 -> [w284]
          tunnel: [w283] -> w278
          tunnel: w277 -> [w283]
          tunnel: w280 -> [w290]
          tunnel: w278 -> [w287]
          frame #0 {
            n200 = property on="曲线模型" class="Clust (严格)"() -> ("Value"=w282:T2)  [unwired: 2 in, 2 out]
            n201 = call "曲线模型计算.vi"("曲线模型"=w282) -> ("输出簇"=w281:T2)  [unwired: 10 in]
            n202 = property on="曲线模型" class="Clust (严格)"("Value"=w281) -> ()  [unwired: 2 in, 2 out]
          }
          frame #1 {
            n203 = property class="Enum (严格)"(reference=w287) -> ("Value"=w286:enum16{"低量程", "高量程"})  [unwired: 1 in, 2 out]
            n204 = property class="Ring (严格)"(reference=w290) -> ("Value"=w289:u16)  [unwired: 1 in, 2 out]
            n205 = call "id参数转换.vi"("id"=w289) -> ("table输出"=w288:string)  [unwired: 9 in, 1 out]
            n206 = property on="曲线模型" class="Clust (严格)"() -> ("Value"=w285:T2)  [unwired: 2 in, 2 out]
            n207 = case shown="\"氨氮\"" w288 {
              tunnel: w285 -> [_ w292 w298 w301 w304 w308 w312 w316 w320 w325]
              tunnel: w286 -> [_ w291 w295 w299 w303 w307 w311 w315 w319 w323]
              frame Default {
              }
              frame "总磷" {
                n208 = global read "校准数据全局变量.vi" "总磷曲线模型"() -> (w293:T7)
                n209 = Replace Array Subset(array=w293, new element=w292, index=w291) -> (w294:T7)
                n210 = global write "校准数据全局变量.vi" "总磷曲线模型"(w294) -> ()
              }
              frame "总氮" {
                n211 = global read "校准数据全局变量.vi" "总氮曲线模型"() -> (w297:T7)
                n212 = Replace Array Subset(array=w297, new element=w298, index=w295) -> (w296:T7)
                n213 = global write "校准数据全局变量.vi" "总氮曲线模型"(w296) -> ()
              }
              frame "氨氮" {
                n214 = global read "校准数据全局变量.vi" "氨氮曲线模型"() -> (w302:T7)
                n215 = Replace Array Subset(array=w302, new element=w301, index=w299) -> (w300:T7)
                n216 = global write "校准数据全局变量.vi" "氨氮曲线模型"(w300) -> ()
              }
              frame "磷酸盐" {
                n217 = global read "校准数据全局变量.vi" "磷酸盐曲线模型"() -> (w306:T7)
                n218 = Replace Array Subset(array=w306, new element=w304, index=w303) -> (w305:T7)
                n219 = global write "校准数据全局变量.vi" "磷酸盐曲线模型"(w305) -> ()
              }
              frame "硝氮" {
                n220 = global read "校准数据全局变量.vi" "硝氮曲线模型"() -> (w310:T7)
                n221 = Replace Array Subset(array=w310, new element=w308, index=w307) -> (w309:T7)
                n222 = global write "校准数据全局变量.vi" "硝氮曲线模型"(w309) -> ()
              }
              frame "亚硝氮" {
                n223 = global read "校准数据全局变量.vi" "亚硝氮曲线模型"() -> (w314:T7)
                n224 = Replace Array Subset(array=w314, new element=w312, index=w311) -> (w313:T7)
                n225 = global write "校准数据全局变量.vi" "亚硝氮曲线模型"(w313) -> ()
              }
              frame "硅酸盐" {
                n226 = global read "校准数据全局变量.vi" "硅酸盐曲线模型"() -> (w318:T7)
                n227 = Replace Array Subset(array=w318, new element=w316, index=w315) -> (w317:T7)
                n228 = global write "校准数据全局变量.vi" "硅酸盐曲线模型"(w317) -> ()
              }
              frame "硫化物" {
                n229 = global read "校准数据全局变量.vi" "硫化物曲线模型"() -> (w322:T7)
                n230 = Replace Array Subset(array=w322, new element=w320, index=w319) -> (w321:T7)
                n231 = global write "校准数据全局变量.vi" "硫化物曲线模型"(w321) -> ()
              }
              frame "CODcr" {
                n232 = global read "校准数据全局变量.vi" "CODcr曲线模型"() -> (w326:T7)
                n233 = Replace Array Subset(array=w326, new element=w325, index=w323) -> (w324:T7)
                n234 = global write "校准数据全局变量.vi" "CODcr曲线模型"(w324) -> ()
              }
            }
          }
          frame #2 {
            n235 = call "校准数据写入配置文件.vi"() -> ()  [unwired: 11 in, 1 out]
          }
        }
        n236 = Format Date/Time String() -> (date/time string=→"刷新时间":string)  [unwired: 3 in]
      }
      event "校准按钮": Value Change {
        n237 = event-data() -> ("NewVal"=w329:T1)  [unwired: 1 in, 5 out]
        n238 = Not Equal?(x=w329, y=T1."未选择") -> (x != y?=w330:bool)
        n239 = case shown="真" w330 {
          tunnel: w334 -> [_ _]
          tunnel: w333 -> [_ w344]
          tunnel: w332 -> [_ w343]
          tunnel: w329 -> [_ w339]
          tunnel: w328 -> [_ _]
          tunnel: w327 -> [_ w342]
          frame False {
          }
          frame True {
            w336 = T4 {"id"=1, "任务类型"=enum."未选择", "量程下拉列表"=enum."低量程", "状态"=enum."待执行", "标液浓度"=0.0, "吸光值"=0.0, "校准时间"=timestamp(0 s since 1904-01-01)}  # 校准任务
            n240 = property class="Enum (严格)"(reference=w343) -> ("Value"=w340:enum16{"低量程", "高量程"})  [unwired: 1 in, 2 out]
            n241 = property class="Ring (严格)"(reference=w344) -> ("Value"=w341:u16)  [unwired: 1 in, 2 out]
            n242 = property on="曲线模型" class="Clust (严格)"() -> ("Value"=w338:T2)  [unwired: 2 in, 2 out]
            n243 = case shown="\"未选择\", 默认" w339 {
              tunnel: w338 -> [_ w346 w348 w350 w352 w354]
              tunnel: [_ w345 w347 w349 w351 w353] -> w337
              frame "未选择", Default {
              }
              frame "空白校准" {
                n244 = Unbundle By Name(w346) -> ("标液浓度1"=w345:dbl)
              }
              frame "标样校准" {
                n245 = Unbundle By Name(w348) -> ("标液浓度2"=w347:dbl)
              }
              frame "标样核查" {
                n246 = Unbundle By Name(w350) -> ("标液浓度3"=w349:dbl)
              }
              frame "零点核查" {
                n247 = Unbundle By Name(w352) -> ("标液浓度4"=w351:dbl)
              }
              frame "跨度核查" {
                n248 = Unbundle By Name(w354) -> ("标液浓度5"=w353:dbl)
              }
            }
            n249 = Bundle By Name(cluster=w336, "id"=w341, "任务类型"=w339, "量程下拉列表"=w340, "标液浓度"=w337) -> (w335:T4)
            n250 = Generate User Event(user event=w342, event data cluster=w335) -> ()  [unwired: 2 in, 2 out]
          }
        }
      }
      event "历史数据导入": Value Change {
        n251 = event-data() -> ("NewVal"=w357:T1)  [unwired: 1 in, 5 out]
        n252 = Not Equal?(x=w357, y=T1."未选择") -> (x != y?=w358:bool)
        n253 = case shown="真" w358 {
          tunnel: w362 -> [_ _]
          tunnel: w361 -> [_ w372]
          tunnel: w360 -> [_ w365]
          tunnel: w357 -> [_ w363]
          tunnel: w356 -> [_ _]
          tunnel: w355 -> [_ w367]
          frame False {
          }
          frame True {
            n254 = property class="Enum (严格)"(reference=w365) -> ("Value"=w364:enum16{"低量程", "高量程"})  [unwired: 1 in, 2 out]
            n255 = property class="Ring (严格)"(reference=w372) -> ("Value"=w366:u16)  [unwired: 1 in, 2 out]
            n256 = call "id参数转换.vi"("id"=w366) -> ("table输出"=w371:string)  [unwired: 9 in, 1 out]
            n257 = property on="历史数据导入" class="RadioBtnsControl (严格)"("Value"=T1."未选择" ("历史数据导入")) -> ()  [unwired: 2 in, 2 out]
            n258 = call "校准数据选择表.vi"("测量模式"=w363, "量程下拉列表"=w364, "table"=w371) -> ("布尔"=w370:bool, "输出"=w369:T11)  [unwired: 7 in]
            n259 = case shown="真" w370 {
              tunnel: w369 -> [_ w380]
              tunnel: w363 -> [_ w382]
              tunnel: w367 -> [_ w381]
              tunnel: w366 -> [_ w379]
              tunnel: w364 -> [_ w378]
              frame False {
              }
              frame True {
                w376 = T4 {"id"=1, "任务类型"=enum."未选择", "量程下拉列表"=enum."低量程", "状态"=enum."已执行", "标液浓度"=0.0, "吸光值"=0.0, "校准时间"=timestamp(0 s since 1904-01-01)}  # 校准任务
                n260 = Unbundle By Name(w380) -> ("标液值"=w373:dbl, "吸光值"=w374:dbl, "时间"=w375:timestamp)
                n261 = Bundle By Name(cluster=w376, "id"=w379, "任务类型"=w382, "量程下拉列表"=w378, "标液浓度"=w373, "吸光值"=w374, "校准时间"=w375) -> (w377:T4)
                n262 = Generate User Event(user event=w381, event data cluster=w377) -> ()  [unwired: 2 in, 2 out]
              }
            }
          }
        }
      }
      event "校准任务": Value Change {
        n263 = event-data() -> ("NewVal"=w383:bool)  [unwired: 1 in, 5 out]
        n264 = invoke on="子面板" class="SubPnl" method="Remove VI"() -> (error out=w385:errorcluster)  [unwired: 3 in, 2 out]
        n265 = case shown="真" w383 {
          tunnel: w385 -> [_ w392]
          tunnel: w384 -> [_ w389]
          frame False {
          }
          frame True {
            n266 = vi-ref "校准任务设置.vi"() -> (w391:refnum<vi>)
            n267 = property class="VI"(reference=w391) -> (reference out=w387:refnum<vi>, "Name"=w390:string, "Exec.State"=w388:T12)  [unwired: 1 in, 1 out]
            n268 = case shown="\"Idle\"" w388 {
              tunnel: w390 -> [_ w404]
              tunnel: w389 -> [_ w401]
              tunnel: [w393 w397] -> w386
              tunnel: w387 -> [w393 w397]
              frame "Bad", Default {
              }
              frame "Idle" {
                n269 = Open VI Reference(type specifier VI Refnum (for type only)=refnum<vi> refnum, vi path=w404, options=128 ("选项")) -> (vi reference=w402:refnum<vi>, error out=w399:errorcluster)  [unwired: 3 in]
                n270 = property on="模型" class="Enum (严格)"() -> ("Value"=w395:enum32{"线性", "多项式"})  [unwired: 2 in, 2 out]
                n271 = property on="精度" class="DigNum (严格)"() -> ("Value"=w394:dbl)  [unwired: 2 in, 2 out]
                n272 = call-by-ref "开始异步调用"(reference=w402, error in=w399, "精度"=w394, "模型"=w395, "用户事件"=w401) -> (reference out=w400:refnum<vi>, error out=w398:errorcluster)  [unwired: 9 in]
                n273 = Close Reference(reference=w400, error in (no error)=w398) -> ()  [unwired: 1 out]
              }
            }
            n274 = invoke on="子面板" class="SubPnl" method="Insert VI"(error in=w392, "VI Ref"=w386) -> ()  [unwired: 2 in, 4 out]
          }
        }
      }
    }
  }
